vi "from_json.vi"(8 "error in":errorcluster, 10 "json":string, 11 "properties in":refnum<class "properties.lvclass">) -> (0 "error out":errorcluster, 3 "properties out":refnum<class "properties.lvclass">)   [LabVIEW 2020, in "nominal types.lvlib" / "properties.lvclass"]
uses:
  properties.lvclass
  properties.lvclass/properties.ctl
  <vilib>/JDP Science/JSONtext/JSONtext.lvlib
  0b6facf3-7b7a-47ad-9322-a02dd5dd4c91.vi
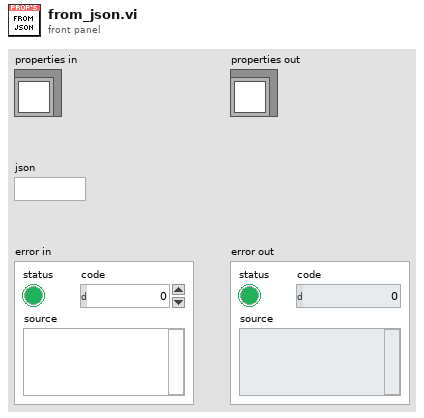
[diagram p1: front panel]
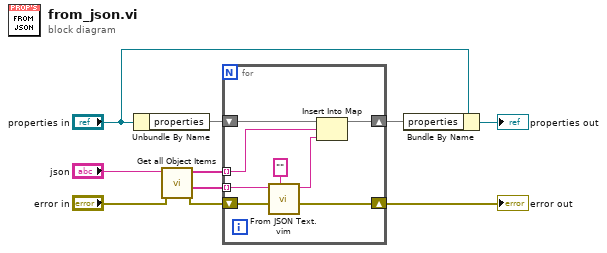
[diagram p0: block diagram]
diagram:
  n1 = Unbundle By Name("properties in") -> ("properties"=w7:map{string, string})
  n2 = call <vilib>:"Get all Object Items.vi"("error in (no error)"="error in", "JSON"="json") -> ("error out"=w3:errorcluster, "<JSON>"=w8:string[], "Item Names"=w9:string[])  [unwired: 6 in, 1 out]
  n3 = for {
    tunnel: w9 -> [w17] mode=indexing
    tunnel: w8 -> [w15] mode=indexing
    shift-right: [w16] -> w5
    shift-left: w7 -> [w18]
    shift-right: [w11] -> w1
    shift-left: w3 -> [w12]
    n4 = call "From JSON Text.vim"("Data Type and Default Value"="", "error in (no error)"=w12, "JSON"=w15) -> ("error out"=w11:errorcluster, "Data out"=w13:string)  [unwired: 7 in]
    n5 = Insert Into Map(map in=w18, key=w17, value=w13) -> (map out=w16:map{string, string})  [unwired: 2 out]
  }
  "error out" <- w1
  n6 = Bundle By Name(cluster="properties in", "properties"=w5) -> (→"properties out":refnum<class "properties.lvclass">)
